vi "Prime BSI Sort File Names.vi"(7 "Requested File Path":path) -> (8 "Resulting File Path":path)   [LabVIEW 2016]
uses:
  kernel32.dll
  shell32.dll
panel:
  out "ReName Success?":bool
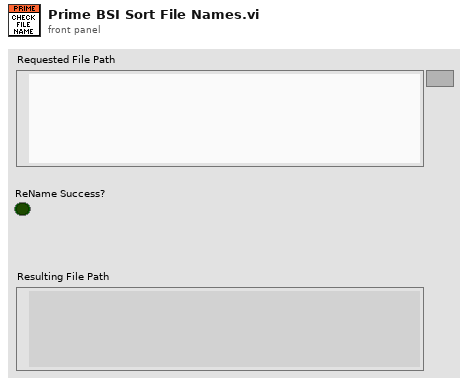
[diagram p1: front panel]
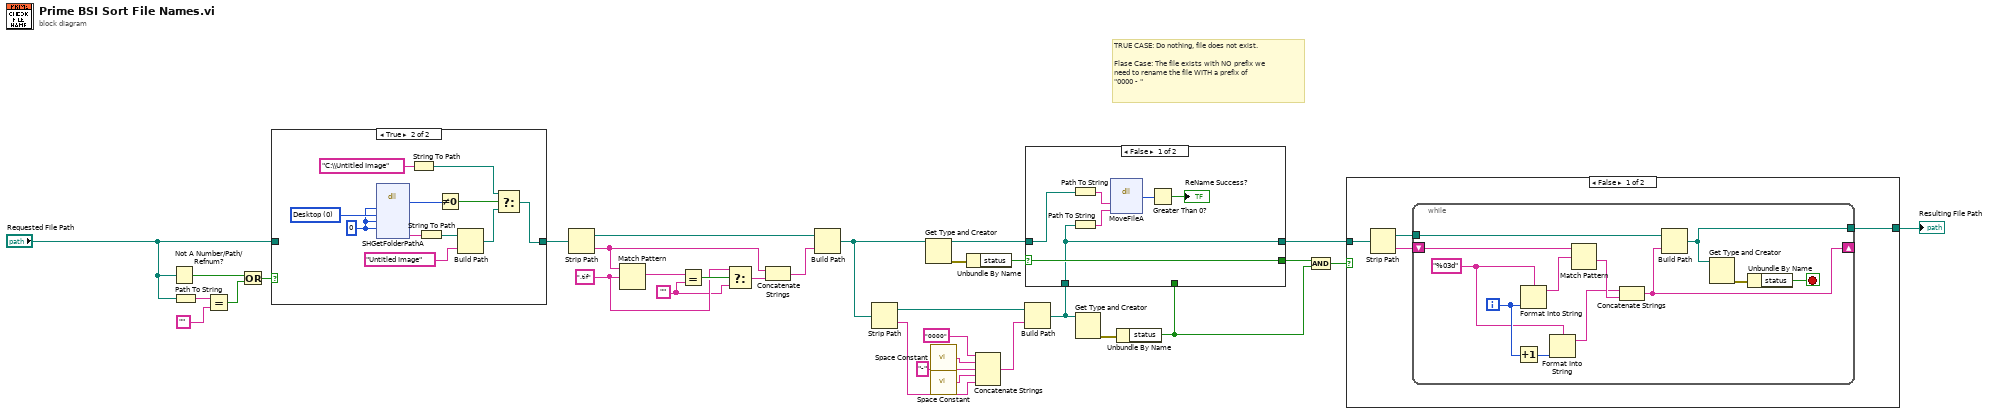
[diagram p0: block diagram]
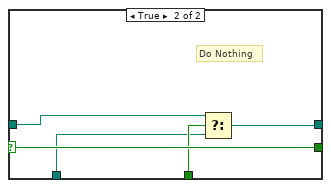
[diagram p3: hidden frame]
diagram:
  w11 = ""
  w12 = ".tif" ("regular expression")
  # "TRUE CASE: Do nothing, file does not exist.\n\nFlase Case: The file exists with NO prefix we\nneed to rename the file WITH a prefix of\n\"0000 - \""
  n1 = Not A Number/Path/Refnum?(number/path/refnum="Requested File Path") -> (NaN/Path/Refnum?=w5:bool)
  n2 = Path To String(path="Requested File Path") -> (string=w7:string)
  n3 = Equal?(x=w7, y="") -> (x = y?=w4:bool)
  n4 = Or(x=w5, y=w4) -> (x .or. y?=w3:bool)
  n5 = case shown="True" w3 {
    tunnel: "Requested File Path" -> [w34 _]
    tunnel: [w34 w35] -> w1
    frame False {
    }
    frame True {
      w45 = 0 items=["Desktop"=0, "Personal Documents"=5, "AppData"=26, "Local AppData"=28, "Common AppData"=35, "Program Files"=38, "Program Files Common"=43, "Common Documents"=46] ("Requested Path")
      w44 = 0 ("HWND")
      n6 = dll-call lib="shell32.dll" fn="SHGetFolderPathA"("HWND"=w44, "nFolder"=w45, "hToken"=w44, "dwFlags"=w44) -> ("Succeeded"=w40:i32, "pszPath"=w43:string)  [unwired: 8 in, 2 out]
      n7 = String To Path(string="C:\\Untitled Image" ("regular expression")) -> (path=w37:path)
      n8 = String To Path(string=w43) -> (path=w42:path)
      n9 = Not Equal To 0?(x=w40) -> (x != 0?=w38:bool)
      n10 = Build Path(base path=w42, name or relative path="Untitled Image" ("regular expression")) -> (appended path=w36:path)
      n11 = Select(t=w37, s=w38, f=w36) -> (s? t:f=w35:path)
    }
  }
  n12 = Strip Path(path=w1) -> (stripped path=w8:path, name=w13:string)
  n13 = Match Pattern(string=w13, regular expression=w12) -> (match substring=w16:string)  [unwired: 1 in, 3 out]
  n14 = Equal?(x=w16, y=w11) -> (x = y?=w15:bool)
  n15 = Select(t=w12, s=w15, f=w11) -> (s? t:f=w14:string)
  n16 = Concatenate Strings(w13, w14) -> (w9:string)
  n17 = Build Path(base path=w8, name or relative path=w9) -> (appended path=w10:path)
  n18 = Strip Path(path=w10) -> (stripped path=w29:path, name=w25:string)
  n19 = Get Type and Creator(7:w10) -> (0:w32:errorcluster, 3:w20:path)  [unwired: 1 in, 2 out]
  n20 = call <vilib>:"Space Constant.vi"() -> ("String"=w31:string)
  n21 = call <vilib>:"Space Constant.vi"() -> ("String"=w27:string)
  n22 = Unbundle By Name(w32) -> ("status"=w22:bool)
  n23 = Concatenate Strings("0000", w31, "-", w27, w25) -> (w28:string)
  n24 = Build Path(base path=w29, name or relative path=w28) -> (appended path=w18:path)
  n25 = Get Type and Creator(7:w18) -> (0:w24:errorcluster)  [unwired: 1 in, 3 out]
  n26 = Unbundle By Name(w24) -> ("status"=w17:bool)
  n27 = case shown="False" w22 {
    selector: w22 -> [w52 w57]
    tunnel: [w52 w57] -> w21
    tunnel: w20 -> [w47 w55]
    tunnel: [w46 w54] -> w19
    tunnel: w18 -> [w46 w53]
    tunnel: w17 -> [_ w56]
    frame False {
      n28 = Path To String(path=w47) -> (string=w49:string)
      n29 = Path To String(path=w46) -> (string=w48:string)
      n30 = dll-call lib="kernel32.dll" fn="MoveFileA"(w49, w48) -> ("return type"=w50:i32)  [unwired: 5 in, 2 out]
      n31 = Greater Than 0?(x=w50) -> (x > 0?=→"ReName Success?":bool)
    }
    frame True {
      # "Do Nothing"
      n32 = Select(t=w55, s=w56, f=w53) -> (s? t:f=w54:path)
    }
  }
  n33 = And(x=w21, y=w17) -> (x .and. y?=w23:bool)
  n34 = case shown="False" w23 {
    tunnel: w19 -> [w61 w74]
    tunnel: [w58 w74] -> w33
    frame False {
      n35 = Strip Path(path=w61) -> (stripped path=w60:path, name=w59:string)
      n36 = while {
        tunnel: w60 -> [w72]
        tunnel: [w69] -> w58
        shift-right: [w62] -> _
        shift-left: w59 -> [w73]
        i -> [w66]
        stop <- w67 stop-if-true
        w64 = "%03d" ("format string")
        n37 = Increment(x=w66) -> (x+1=w65:i32)
        n38 = Format Into String(format string=w64, w66) -> (resulting string=w71:string)  [unwired: 2 in, 1 out]
        n39 = Format Into String(format string=w64, w65) -> (resulting string=w63:string)  [unwired: 2 in, 1 out]
        n40 = Match Pattern(string=w73, regular expression=w71) -> (after substring=w70:string)  [unwired: 1 in, 3 out]
        n41 = Concatenate Strings(w63, w70) -> (w62:string)
        n42 = Build Path(base path=w72, name or relative path=w62) -> (appended path=w69:path)
        n43 = Get Type and Creator(7:w69) -> (0:w68:errorcluster)  [unwired: 1 in, 3 out]
        n44 = Unbundle By Name(w68) -> ("status"=w67:bool)
      }
    }
    frame True {
      # "File does NOT exist - Do NOTHING"
    }
  }
  "Resulting File Path" <- w33
